vi "Declare Dependency.vi"(6 "Shared Resource (F)":bool, 7 "Dependency":refnum<class "Dependency.lvclass">, 8 "error in (no error)":errorcluster, 9 "Start Order (0)":i8, 10 "Name":string, 11 "Type":refnum<class "SMO.lvclass">) -> (0 "error out":errorcluster, 3 "Dependency out":refnum<class "Dependency.lvclass">)   [LabVIEW 2021, in "smo.lvlib" / "Dependency.lvclass"]
uses:
  Dependency.lvclass
  SMO/SMO.lvclass
  Dependency.lvclass/Dependency.ctl
  <vilib>/regexp/Match Regular Expression.xnode
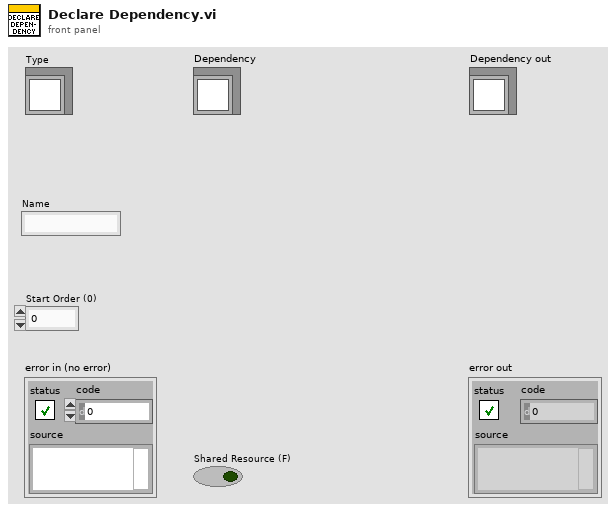
[diagram p1: front panel]
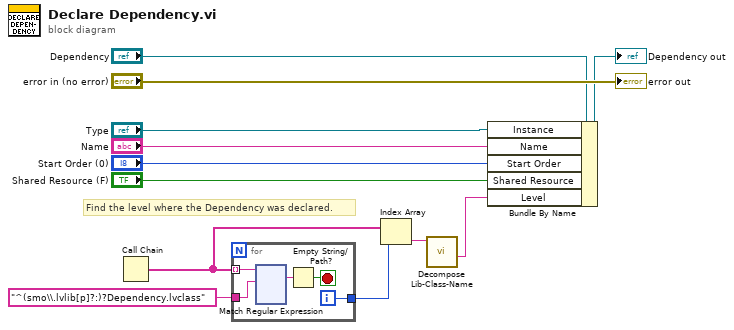
[diagram p0: block diagram]
diagram:
  # "Find the level where the Dependency was declared."
  n1 = Call Chain() -> (call chain=w4:string[])
  n2 = for {
    tunnel: w4 -> [w17] mode=indexing
    tunnel: "^(smo\\.lvlib[p]?:)?Dependency.lvclass" -> [w16]
    tunnel: [w13] -> w3
    i -> [w13]
    stop <- w14 stop-if-true
    n3 = xnode "Match Regular Expression"("input string"=w17, "regular expression"=w16) -> ("whole match"=w15:string)  [unwired: 4 in, 4 out]
    n4 = Empty String/Path?(string/path=w15) -> (empty?=w14:bool)
  }
  n5 = Index Array(array=w4, index=w3) -> (element=w1:string)
  n6 = call "Decompose Lib-Class-Name.vi"("Qualified Name"=w1) -> ("className"=w2:string)  [unwired: 6 in, 4 out]
  n7 = Bundle By Name(cluster="Dependency", "Instance"="Type", "Name"="Name", "Start Order"="Start Order (0)", "Shared Resource"="Shared Resource (F)", "Level"=w2) -> (→"Dependency out":refnum<class "Dependency.lvclass">)
  "error out" <- "error in (no error)"
